vi "pulse_generator_data_daqmx.vi"(8 "error in":errorcluster, 10 "Pulse Generator Input Physical Channels":T1={"Absolute Pressure"="cDAQ1Mod5/ai20", "PG to TS dP"="cDAQ1Mod5/cDAQ1Mod5/ai21", "Pitot dP"="cDAQ1Mod8/ai8", "PG Temperature 1"="cDAQ1Mod6/ai4", "PG Temperature 2"="cDAQ1Mod6/ai5", "dP Windows 1 to 7"="cDAQ1Mod8/ai11", "dP Windows 1 to 4"="cDAQ1Mod8/ai10", "Camera Voltage"="cDAQ1Mod2/ai0", "dP Windows 1 to 4 F"="cDAQ1Mod2/ai0"}, 11 "task in":refnum<k21>) -> (0 "error out":errorcluster, 3 "task out":refnum<k21>)   [LabVIEW 2017]
uses:
  Input Channel Lists/pulse_generator_input_physical_channels.ctl
  <vilib>/DAQmx/create/channels.llb/DAQmx Create Channel (AI-Voltage-Basic).vi
  <vilib>/DAQmx/create/channels.llb/DAQmx Create Channel (AI-Current-Basic).vi
  <vilib>/DAQmx/create/channels.llb/DAQmx Create Channel (AI-Temperature-Thermocouple).vi
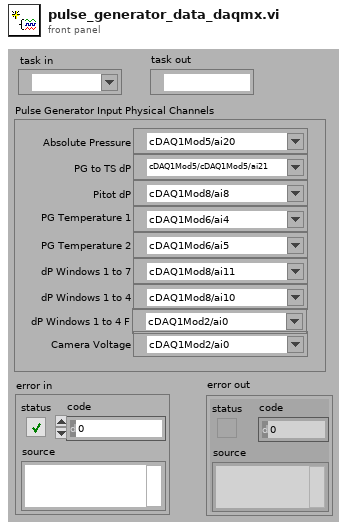
[diagram p1: front panel]
types:
  T1 = typedef "pulse_generator_input_physical_channels.ctl" = cluster{"Absolute Pressure":tag, "PG to TS dP":tag, "Pitot dP":tag, "PG Temperature 1":tag, "PG Temperature 2":tag, "dP Windows 1 to 7":tag, "dP Windows 1 to 4":tag, "Camera Voltage":tag, "dP Windows 1 to 4 F":tag}
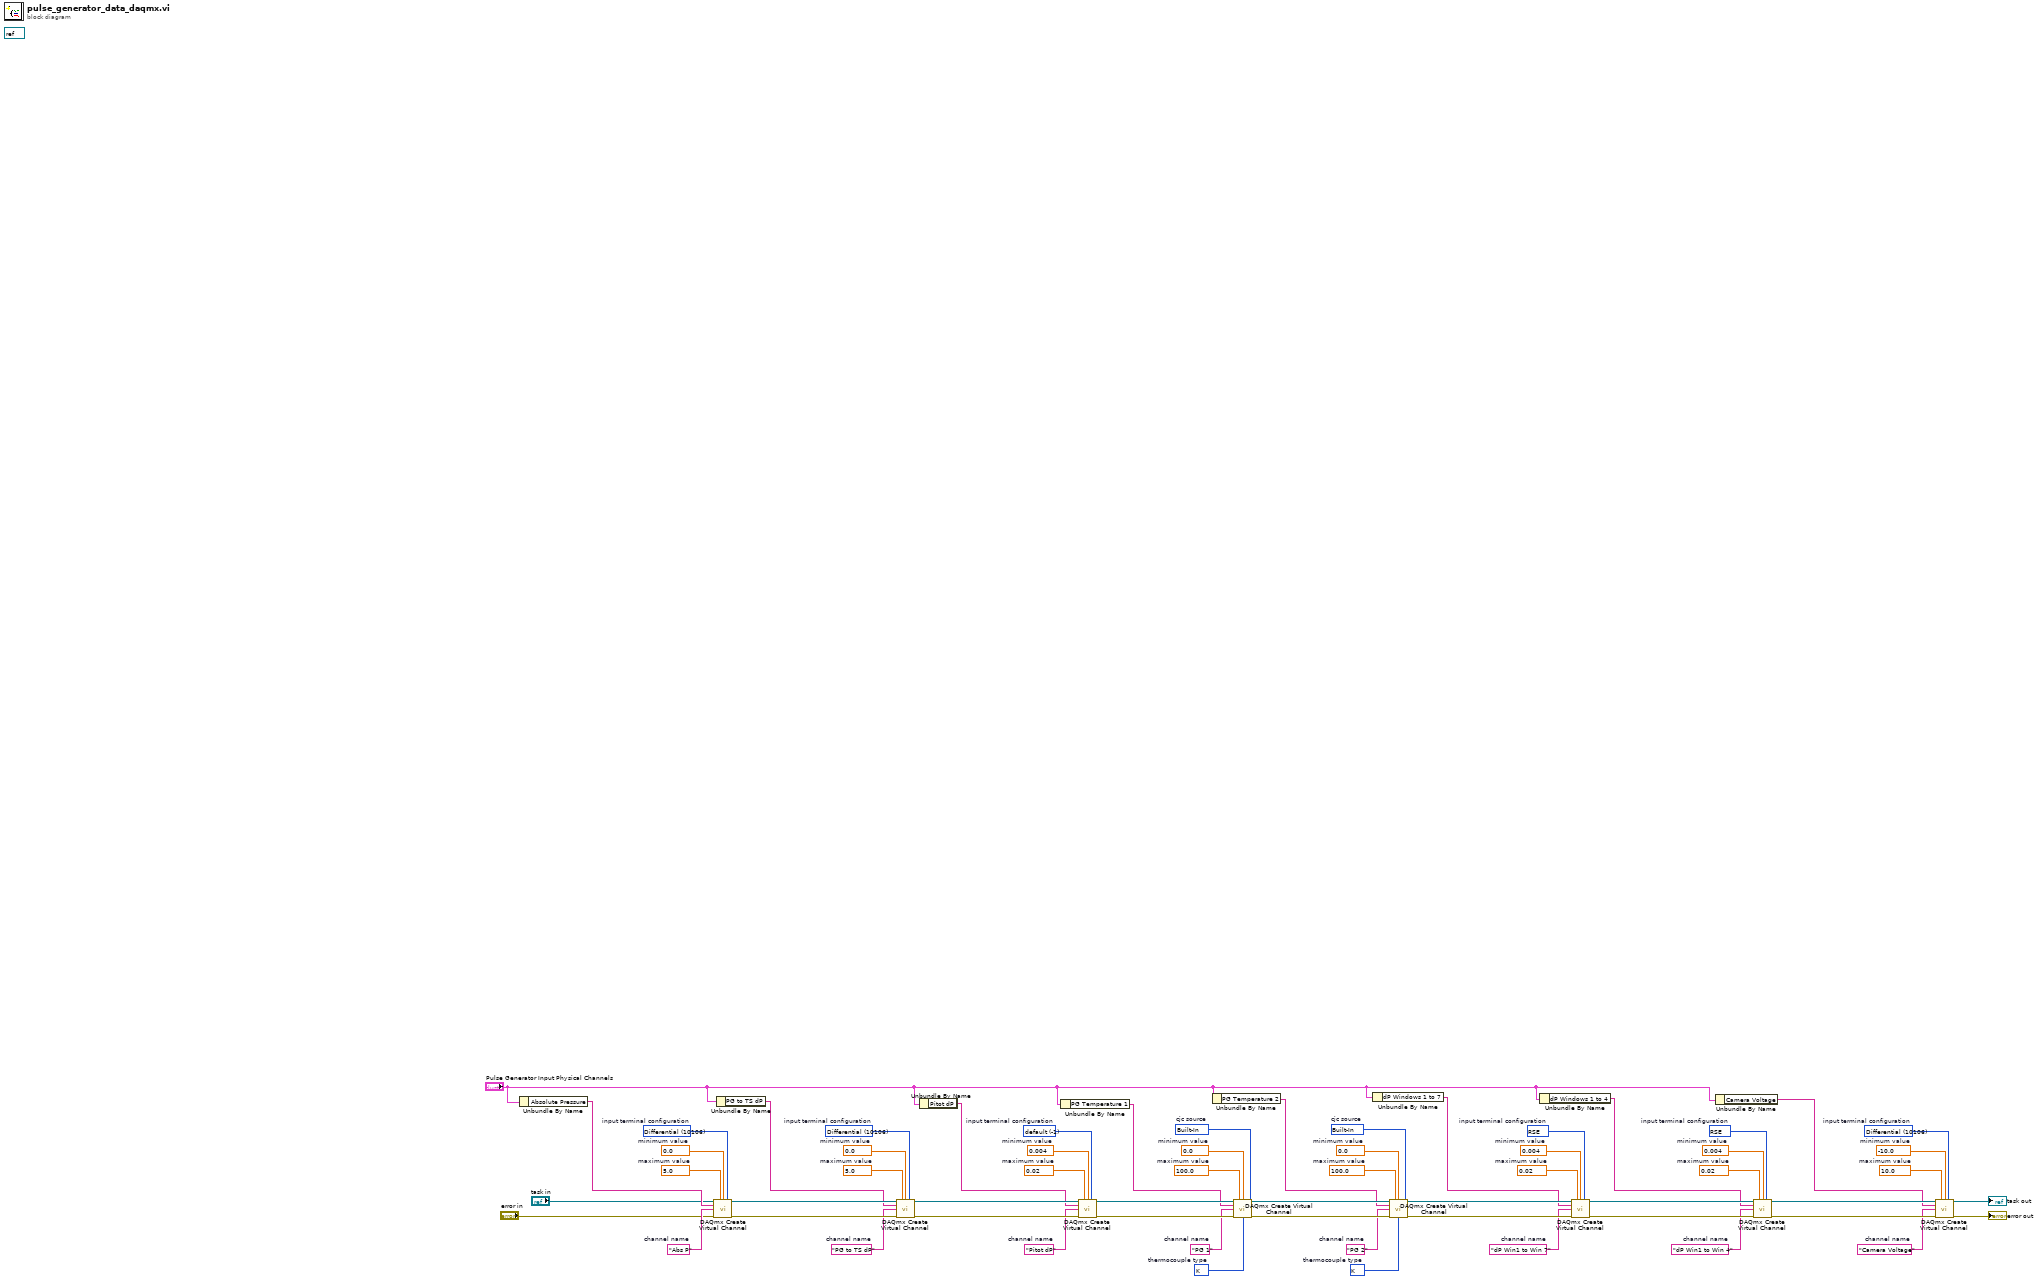
[diagram p0: block diagram]
diagram:
  (unwired) refnum<k21> refnum ("task out")
  w14 = 10106 items=["default"=-1, "RSE"=10083, "NRSE"=10078, "Differential"=10106, "Pseudodifferential"=12529]  # input terminal configuration
  w15 = "Camera Voltage"  # channel name
  w16 = -10.0  # minimum value
  w17 = 10.0  # maximum value
  w19 = 10083 items=["default"=-1, "RSE"=10083, "NRSE"=10078, "Differential"=10106, "Pseudodifferential"=12529]  # input terminal configuration
  w20 = "dP Win1 to Win 4"  # channel name
  w22 = 0.004  # minimum value
  w23 = 0.02  # maximum value
  w25 = 10083 items=["default"=-1, "RSE"=10083, "NRSE"=10078, "Differential"=10106, "Pseudodifferential"=12529]  # input terminal configuration
  w26 = "dP Win1 to Win 7"  # channel name
  w28 = 0.004  # minimum value
  w29 = 0.02  # maximum value
  w31 = 10200 items=["Built-In"=10200, "Constant Value"=10116, "Channel"=10113]  # cjc source
  w33 = 10073 items=["J"=10072, "K"=10073, "N"=10077, "R"=10082, "S"=10085, "T"=10086, "B"=10047, "E"=10055]  # thermocouple type
  w32 = "PG 2"  # channel name
  w35 = 0.0  # minimum value
  w36 = 100.0  # maximum value
  w38 = 10200 items=["Built-In"=10200, "Constant Value"=10116, "Channel"=10113]  # cjc source
  w40 = 10073 items=["J"=10072, "K"=10073, "N"=10077, "R"=10082, "S"=10085, "T"=10086, "B"=10047, "E"=10055]  # thermocouple type
  w39 = "PG 1"  # channel name
  w42 = 0.0  # minimum value
  w43 = 100.0  # maximum value
  w45 = -1 items=["default"=-1, "RSE"=10083, "NRSE"=10078, "Differential"=10106, "Pseudodifferential"=12529]  # input terminal configuration
  w46 = "Pitot dP"  # channel name
  w48 = 0.004  # minimum value
  w49 = 0.02  # maximum value
  w51 = 10106 items=["default"=-1, "RSE"=10083, "NRSE"=10078, "Differential"=10106, "Pseudodifferential"=12529]  # input terminal configuration
  w52 = "PG to TS dP"  # channel name
  w54 = 0.0  # minimum value
  w55 = 5.0  # maximum value
  w57 = 10106 items=["default"=-1, "RSE"=10083, "NRSE"=10078, "Differential"=10106, "Pseudodifferential"=12529]  # input terminal configuration
  w58 = "Abs P"  # channel name
  w60 = 0.0  # minimum value
  w61 = 5.0  # maximum value
  n1 = Unbundle By Name("Pulse Generator Input Physical Channels") -> ("Absolute Pressure"=w13:tag)
  n2 = call-poly <vilib>:"DAQmx Create Virtual Channel.vi"("task in"="task in", "maximum value"=w61, "minimum value"=w60, "input terminal configuration"=w57, "physical channels"=w13, "name to assign"=w58, "error in"="error in") -> ("task out"=w56:refnum<k21>, "error out"=w59:errorcluster)  [unwired: 7 in]
  n3 = Unbundle By Name("Pulse Generator Input Physical Channels") -> ("PG to TS dP"=w12:tag)
  n4 = call-poly <vilib>:"DAQmx Create Virtual Channel.vi"("task in"=w56, "maximum value"=w55, "minimum value"=w54, "input terminal configuration"=w51, "physical channels"=w12, "name to assign"=w52, "error in"=w59) -> ("task out"=w50:refnum<k21>, "error out"=w53:errorcluster)  [unwired: 7 in]
  n5 = Unbundle By Name("Pulse Generator Input Physical Channels") -> ("Pitot dP"=w11:tag)
  n6 = Unbundle By Name("Pulse Generator Input Physical Channels") -> ("PG Temperature 1"=w10:tag)
  n7 = call-poly <vilib>:"DAQmx Create Virtual Channel.vi"("task in"=w50, "maximum value"=w49, "minimum value"=w48, "input terminal configuration"=w45, "physical channels"=w11, "name to assign"=w46, "error in"=w53) -> ("task out"=w44:refnum<k21>, "error out"=w47:errorcluster)  [unwired: 7 in]
  n8 = Unbundle By Name("Pulse Generator Input Physical Channels") -> ("PG Temperature 2"=w9:tag)
  n9 = call-poly <vilib>:"DAQmx Create Virtual Channel.vi"("task in"=w44, "maximum value"=w43, "minimum value"=w42, "physical channels"=w10, "cjc source"=w38, "name to assign"=w39, "error in"=w47, "thermocouple type"=w40) -> ("task out"=w37:refnum<k21>, "error out"=w41:errorcluster)  [unwired: 6 in]
  n10 = Unbundle By Name("Pulse Generator Input Physical Channels") -> ("dP Windows 1 to 7"=w7:tag)
  n11 = call-poly <vilib>:"DAQmx Create Virtual Channel.vi"("task in"=w37, "maximum value"=w36, "minimum value"=w35, "physical channels"=w9, "cjc source"=w31, "name to assign"=w32, "error in"=w41, "thermocouple type"=w33) -> ("task out"=w30:refnum<k21>, "error out"=w34:errorcluster)  [unwired: 6 in]
  n12 = Unbundle By Name("Pulse Generator Input Physical Channels") -> ("dP Windows 1 to 4"=w6:tag)
  n13 = call-poly <vilib>:"DAQmx Create Virtual Channel.vi"("task in"=w30, "maximum value"=w29, "minimum value"=w28, "input terminal configuration"=w25, "physical channels"=w7, "name to assign"=w26, "error in"=w34) -> ("task out"=w24:refnum<k21>, "error out"=w27:errorcluster)  [unwired: 7 in]
  n14 = Unbundle By Name("Pulse Generator Input Physical Channels") -> ("Camera Voltage"=w5:tag)
  n15 = call-poly <vilib>:"DAQmx Create Virtual Channel.vi"("task in"=w24, "maximum value"=w23, "minimum value"=w22, "input terminal configuration"=w19, "physical channels"=w6, "name to assign"=w20, "error in"=w27) -> ("task out"=w18:refnum<k21>, "error out"=w21:errorcluster)  [unwired: 7 in]
  n16 = call-poly <vilib>:"DAQmx Create Virtual Channel.vi"("task in"=w18, "maximum value"=w17, "minimum value"=w16, "input terminal configuration"=w14, "physical channels"=w5, "name to assign"=w15, "error in"=w21) -> ("task out"=→"task out":refnum<k21>, "error out"=→"error out":errorcluster)  [unwired: 7 in]
